vi "Read_Write_measurements_files.vi"() -> ()   [LabVIEW 2022 SP3]
panel:
  out "Waveform Graph":dynamicdata(graph)
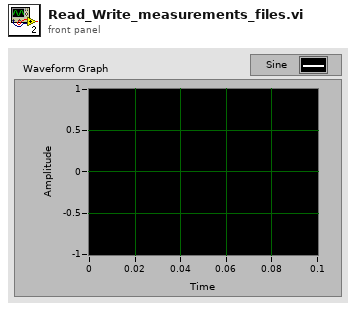
[diagram p1: front panel]
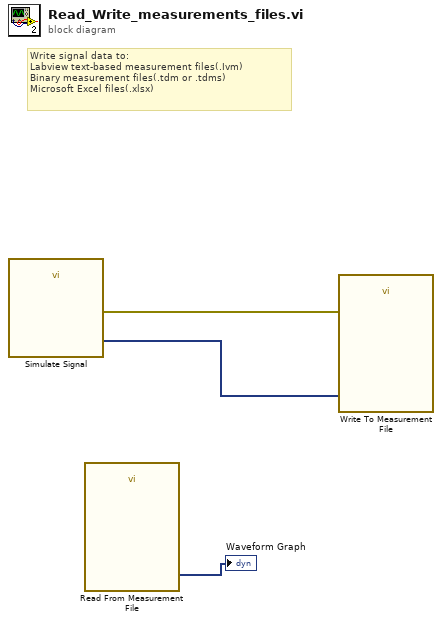
[diagram p0: block diagram]
diagram:
  # "Write signal data to:\nLabview text-based measurement files(.Ivm)\nBinary measurement files(.tdm or .tdms)\nMicrosoft Excel files(.xlsx)"
  n1 = call "Simulate Signal"() -> ("Sine"=w3:dynamicdata, "error out"=w2:errorcluster)  [unwired: 14 in]
  n2 = call "Read From Measurement File"() -> ("Signals"=→"Waveform Graph":dynamicdata)  [unwired: 6 in, 5 out]
  n3 = call "Write To Measurement File"("Signals"=w3, "error in (no error)"=w2) -> ()  [unwired: 15 in, 3 out]
